vi "Update Tree.vi"(8 "Replace?":bool=TRUE, 9 "Tree":T1[](array[typedef]), 10 "Error":errorcluster, 11 "Tree Refnum":refnum<vi>) -> (0 "All Tags":string[](array[string]), 1 "Tree":T1[](array[typedef]), 2 "Error":errorcluster, 3 "Tree Refnum":refnum<vi>)   [LabVIEW 2021, in "Tree.lvlib" / "Tree.lvclass"]
uses:
  Tree.lvclass
  TreeData.ctl
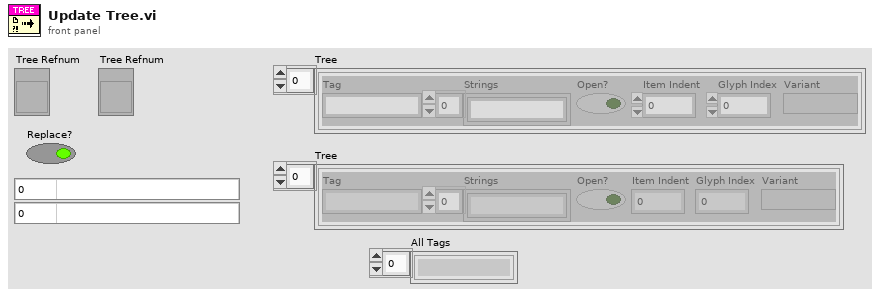
[diagram p1: front panel]
types:
  T1 = typedef "Tree.lvlib/Tree.lvclass/TreeData.ctl" = cluster{"Tag":string, "Strings":string[], "Open?":bool, "Item Indent":i32, "Glyph Index":i32, "Variant":variant}
  T2 = typedef "LVNodeAndColumnTypeDef.ctl" = cluster{"Node":string, "Column":i32}
  T3 = cluster{"Left Cell String":string, "Child Text":string[], "Child Tag":string, "Item Indent":i32, "Child Only?":bool, "Glyph Index":i32}
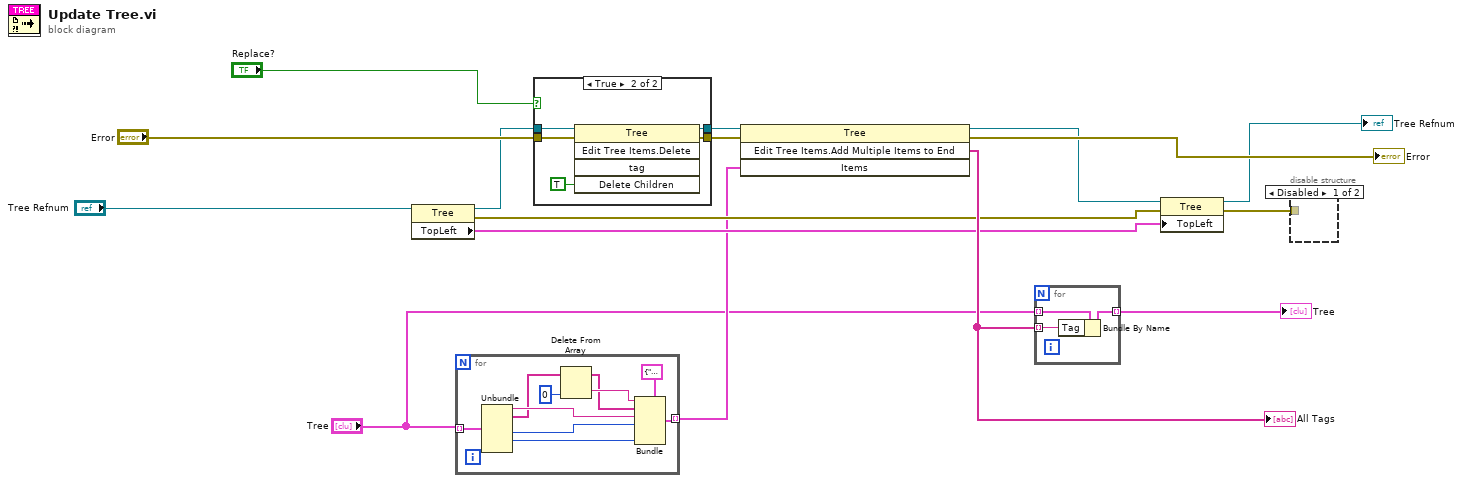
[diagram p0: block diagram]
diagram:
  n1 = property class="Tree"(reference="Tree Refnum") -> (reference out=w6:refnum<vi>, error out=w4:errorcluster, "TopLeft"=w5:T2)  [unwired: 1 in]
  n2 = for {
    tunnel: "Tree" -> [w26] mode=indexing
    tunnel: [w17] -> w2 mode=indexing
    n3 = Unbundle(w26) -> ("Tag"=w24:string, "Strings"=w23:string[], "Item Indent"=w19:i32, "Glyph Index"=w18:i32)  [unwired: 2 out]
    n4 = Delete From Array(array=w23, index=0) -> (deleted portion=w21:string, array with subset deleted=w20:string[])  [unwired: 1 in]
    n5 = Bundle(cluster=T3 {"Left Cell String"="", "Child Text"=[], "Child Tag"="", "Item Indent"=0, "Child Only?"=FALSE, "Glyph Index"=0} ("Item"), "Left Cell String"=w21, "Child Text"=w20, "Child Tag"=w24, "Item Indent"=w19, "Glyph Index"=w18) -> (w17:T3)  [unwired: 1 in]
  }
  n6 = case shown="True" "Replace?" {
    tunnel: [w27 w33] -> w9
    tunnel: [w28 w32] -> w8
    tunnel: "Error" -> [w27 w30]
    tunnel: w6 -> [w28 w29]
    frame False {
    }
    frame True {
      n7 = invoke class="Tree" method="Edit Tree Items.Delete"(reference=w29, error in=w30, "Delete Children"=TRUE ("Delete Children?")) -> (reference out=w32:refnum<vi>, error out=w33:errorcluster)  [unwired: 2 in, 3 out]
    }
  }
  n8 = invoke class="Tree" method="Edit Tree Items.Add Multiple Items to End"(reference=w8, error in=w9, "Items"=w2) -> (reference out=w7:refnum<vi>, error out=→"Error":errorcluster, "Edit Tree Items:Add Multiple Items to End"=w15:string[])  [unwired: 1 in, 1 out]
  "All Tags" <- w15
  n9 = for {
    tunnel: w15 -> [w34] mode=indexing
    tunnel: "Tree" -> [w36] mode=indexing
    tunnel: [w35] -> w10 mode=indexing
    n10 = Bundle By Name(cluster=w36, "Tag"=w34) -> (w35:T1)
  }
  "Tree" <- w10
  n11 = property class="Tree"(reference=w7, error in=w4, "TopLeft"=w5) -> (reference out=→"Tree Refnum":refnum<vi>, error out=w11:errorcluster)
  n12 = disable-structure shown="Disabled" {
    disable-tunnel: w11 -> [_ _]
    frame Disabled {
    }
    frame Enabled {
    }
  }
